vi "plotting.vi"() -> ()   [LabVIEW 2021]
panel:
  in  "Sampling time (sec.)":dbl
  out "Numeric":dbl
  out "Waveform Chart":dbl(graph)
  in  "Stop Button":bool
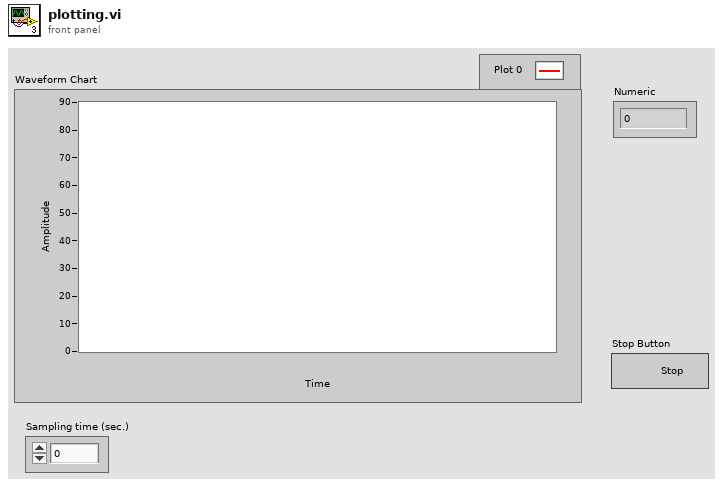
[diagram p1: front panel]
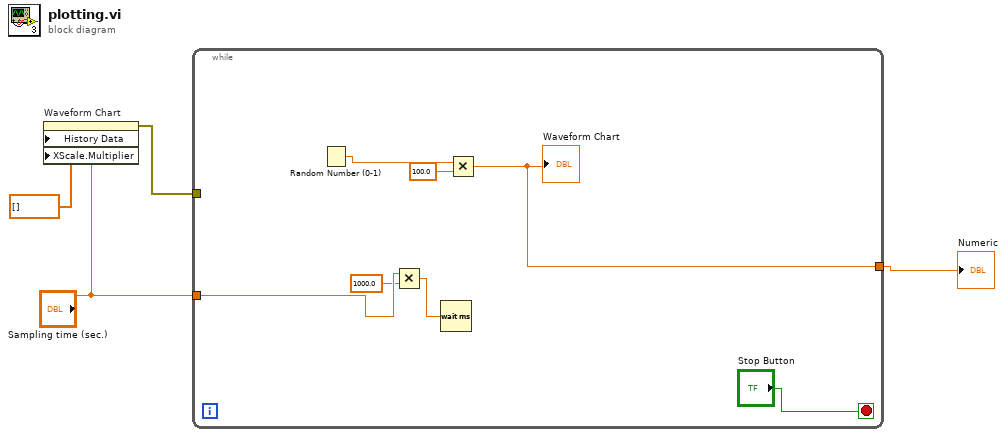
[diagram p0: block diagram]
diagram:
  n1 = property on="Waveform Chart" class="WFChart (strict)"("History Data"=dbl[] [], "XScale.Multiplier"="Sampling time (sec.)") -> (error out=w2:errorcluster)  [unwired: 2 in, 1 out]
  n2 = while {
    tunnel: [w8] -> w4
    tunnel: w2 -> [_]
    tunnel: "Sampling time (sec.)" -> [w7]
    stop <- "Stop Button" stop-if-true
    n3 = Random Number (0-1)() -> (number: 0 to 1=w10:dbl)
    n4 = Multiply(x=w7, y=1000.0) -> (x*y=w5:dbl)
    n5 = Wait (ms)(milliseconds to wait=w5) -> ()  [unwired: 1 out]
    n6 = Multiply(x=w10, y=100.0) -> (x*y=w8:dbl)
    "Waveform Chart" <- w8
  }
  "Numeric" <- w4
